vi "Script Custom Device.vi"(8 "error in":errorcluster, 9 "parameters configuration file path":path caption="path to parameters xml", 10 "hardware configuration file path":path, 11 "system definition path in":path) -> (0 "error out":errorcluster, 1 "Ballard MIL-STD 1553 custom device out":T1 format="%.0x", 2 "System Definition":refnum<k24>, 3 "system definition path out":path)   [LabVIEW 2020, in "Logging Loopback.lvclass"]
uses:
  Logging Loopback.lvclass
  <vilib>/NI VeriStand/Custom Device API/Custom Device Item Ref.ctl
  NationalInstruments.VeriStand.SystemDefinitionAPI
  Shared/Device Parameters.ctl
  Shared/Initialization Method.ctl
  niveristand-custom-device-testing-tools/VeriStandTestUtilities/VeriStandTestUtilities.lvlib
  Scripting/Ballard MIL-STD-1553 Scripting.lvlib
  <vilib>/NI VeriStand/Custom Device API/Custom Device API.lvlib
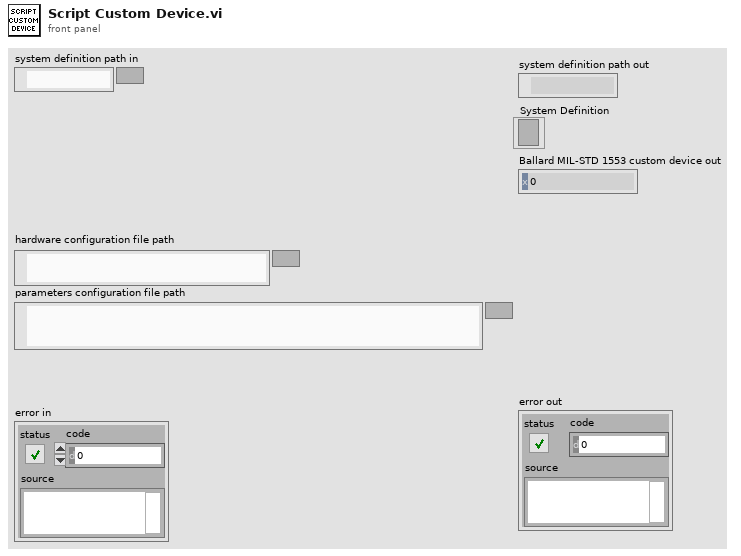
[diagram p1: front panel]
types:
  T1 = typedef "Custom Device API.lvlib/Custom Device Item Ref.ctl" = u64
  T2 = typedef "Device Parameters.ctl" = cluster{"initialization method":T3, "card number":i32, "PXI slot number":i32, "core number":i32}
  T3 = typedef "Initialization Method.ctl" = enum16{"PXI Slot Number", "Card Number"}
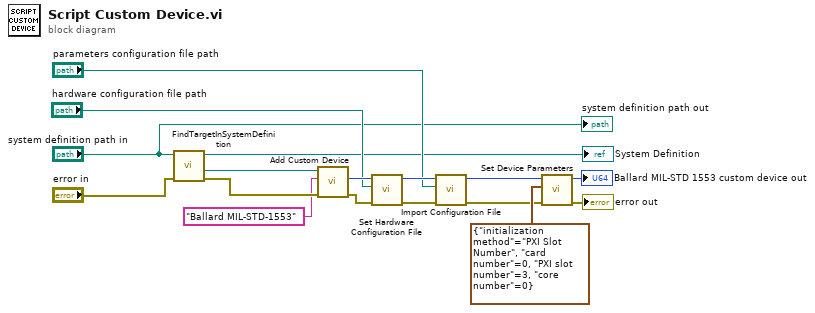
[diagram p0: block diagram]
diagram:
  n1 = call "FindTargetInSystemDefinition.vi"("error in"="error in", "system definition path"="system definition path in") -> ("error out"=w15:errorcluster, "Target"=w13:refnum<k24>, "System Definition"=→"System Definition":refnum<k24>)  [unwired: 6 in, 1 out]
  n2 = call "Add Custom Device.vi"("error in"=w15, "name"="Ballard MIL-STD-1553", "target in"=w13) -> ("error out"=w17:errorcluster, "Ballard MIL-STD 1553 custom device"=w16:T1)  [unwired: 6 in, 1 out]
  n3 = call "Set Hardware Configuration File.vi"("error in"=w17, "hardware configuration file path"="hardware configuration file path", "Ballard MIL-STD 1553 custom device in"=w16) -> ("error out"=w12:errorcluster, "Ballard MIL-STD 1553 custom device out"=w11:T1)  [unwired: 7 in]
  n4 = call "Import Configuration File.vi"("error in"=w12, "parameters configuration file path"="parameters configuration file path", "Ballard MIL-STD 1553 custom device in"=w11) -> ("error out"=w9:errorcluster, "Ballard MIL-STD 1553 custom device out"=w8:T1)  [unwired: 7 in]
  n5 = call "Set Device Parameters.vi"("error in"=w9, "device parameters"=T2 {"initialization method"=enum."PXI Slot Number", "card number"=0, "PXI slot number"=3, "core number"=0}, "Ballard MIL-STD 1553 custom device in"=w8) -> ("error out"=→"error out":errorcluster, "Ballard MIL-STD 1553 custom device out"=→"Ballard MIL-STD 1553 custom device out":T1)  [unwired: 7 in]
  "system definition path out" <- "system definition path in"
